vi "ACP Offset Outer List BW Configure Type.vi"(8 "error in (no error)":errorcluster {"code" format="%.0x"}, 9 "BandwidthType":i32[](array[numeric]), 11 "instrument handle":refnum<k15>) -> (0 "error out":errorcluster {"code" format="%.0x"}, 3 "instrument handle out":refnum<k15>)   [LabVIEW 2021, in "Keysight XSAnVMA.lvlib"]
doc: "Selects a Gaussian filter based on its -3 dB (Normal) bandwidth or its -6 dB bandwidth."
uses:
  <instrlib>/Keysight XSAnVMA/Keysight XSAnVMA.lvlib
  KtXSAnVMA_64.dll
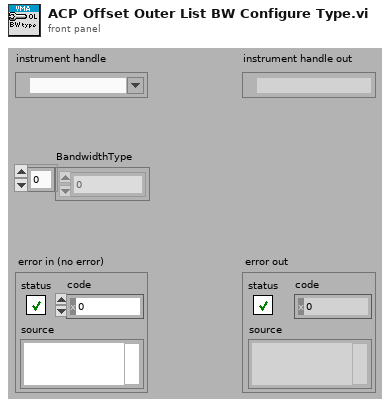
[diagram p1: front panel]
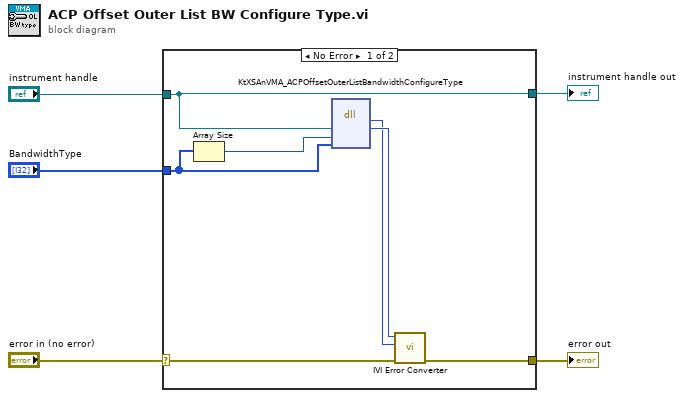
[diagram p0: block diagram]
diagram:
  n1 = case shown="No Error" "error in (no error)" {
    selector: "error in (no error)" -> [w10 w14]
    tunnel: [w9 w14] -> w5
    tunnel: "instrument handle" -> [w8 w13]
    tunnel: "BandwidthType" -> [w7 _]
    tunnel: [w8 w13] -> w1
    frame No Error {
      n2 = Array Size(array=w7) -> (size(s)=w6:i32)
      n3 = dll-call lib="KtXSAnVMA**.dll" fn="KtXSAnVMA_ACPOffsetOuterListBandwidthConfigureType"("Vi"=w8, "BandwidthTypeBufferSize"=w6, "BandwidthType"=w7) -> (w11:i32, "Vi"=w12:u32)  [unwired: 5 in, 2 out]
      n4 = call <instrlib>:"IVI Error Converter.vi"("error in (no error)"=w10, "IVI error code (0)"=w11, "instrument handle"=w12) -> ("error out"=w9:errorcluster)  [unwired: 7 in, 1 out]
    }
    frame Error {
    }
  }
  "error out" <- w5
  "instrument handle out" <- w1
